vi "Zombie.vi"(8 "Error In":errorcluster, 11 "VI In":refnum<vi>) -> (0 "Error Out":errorcluster, 3 "VI Out":refnum<vi>)   [LabVIEW 2017, in "Eulogy.lvlib"]
uses:
  Eulogy.lvlib
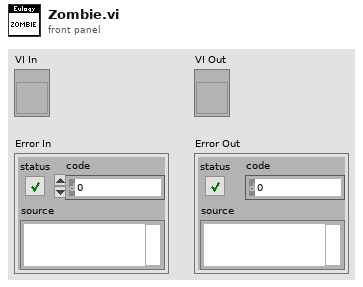
[diagram p1: front panel]
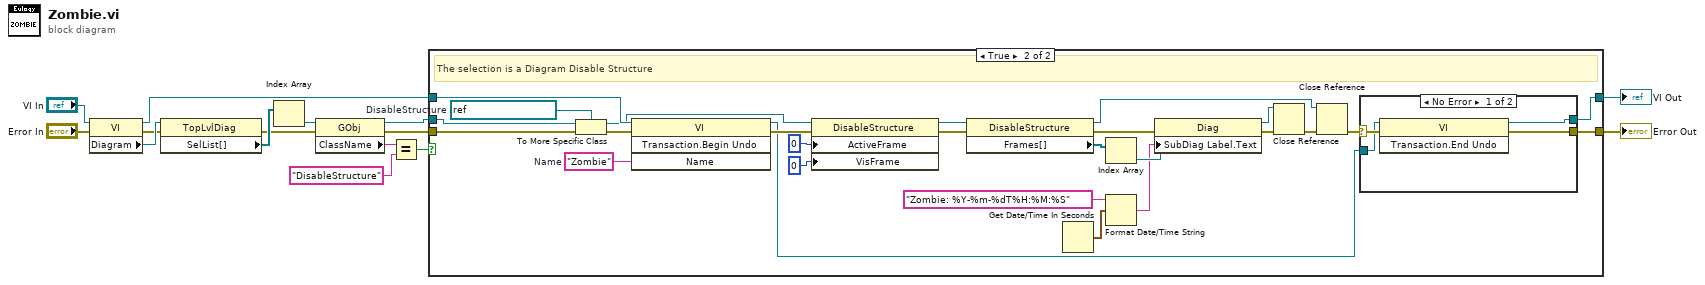
[diagram p0: block diagram]
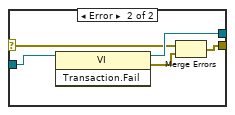
[diagram p3: hidden frame]
diagram:
  n1 = property class="VI"(reference="VI In", error in="Error In") -> (reference out=w7:refnum<vi>, error out=w12:errorcluster, "Diagram"=w13:refnum<vi>)
  n2 = property class="TopLvlDiag"(reference=w13, error in=w12) -> (error out=w9:errorcluster, "SelList[]"=w11:refnum<vi>[])  [unwired: 1 out]
  n3 = Index Array(array=w11) -> (element=w10:refnum<vi>)  [unwired: 1 in]
  n4 = property class="GObj"(reference=w10, error in=w9) -> (reference out=w2:refnum<vi>, error out=w1:errorcluster, "ClassName"=w5:string)
  n5 = Equal?(x=w5, y="DisableStructure") -> (x = y?=w3:bool)
  n6 = case shown="True" w3 {
    tunnel: [w16 w42] -> w15
    tunnel: [w17 w41] -> w14
    tunnel: w7 -> [w17 w40]
    tunnel: w2 -> [_ w38]
    tunnel: w1 -> [w16 w37]
    frame False {
      # "Selection is NOT a grave site, do nothing"
    }
    frame True {
      w39 = refnum<vi> refnum  # DisableStructure
      w43 = "Zombie"  # Name
      # "The selection is a Diagram Disable Structure"
      n7 = To More Specific Class(target class=w39, reference=w38, error in=w37) -> (specific class reference=w34:refnum<vi>, error out=w36:errorcluster)
      n8 = invoke class="VI" method="Transaction.Begin Undo"(reference=w40, error in=w36, "Name"=w43) -> (reference out=w31:refnum<vi>, error out=w35:errorcluster)  [unwired: 1 in, 2 out]
      n9 = property class="DisableStructure"(reference=w34, error in=w35, "ActiveFrame"=i16 0 ("Active Frame"), "VisFrame"=u32 0 ("Visible Frame")) -> (reference out=w29:refnum<vi>, error out=w28:errorcluster)
      n10 = property class="DisableStructure"(reference=w29, error in=w28) -> (reference out=w18:refnum<vi>, error out=w25:errorcluster, "Frames[]"=w27:refnum<vi>[])
      n11 = Get Date/Time In Seconds() -> (seconds since 1Jan1904=w24:timestamp)
      n12 = Index Array(array=w27) -> (element=w26:refnum<vi>)  [unwired: 1 in]
      n13 = Format Date/Time String(time format string (%c)="Zombie: %Y-%m-%dT%H:%M:%S", seconds (now)=w24) -> (date/time string=w22:string)  [unwired: 1 in]
      n14 = property class="Diag"(reference=w26, error in=w25, "SubDiag Label.Text"=w22) -> (reference out=w20:refnum<vi>, error out=w21:errorcluster)
      n15 = Close Reference(reference=w20, error in (no error)=w21) -> (error out=w19:errorcluster)
      n16 = Close Reference(reference=w18, error in (no error)=w19) -> (error out=w30:errorcluster)
      n17 = case shown="No Error" w30 {
        selector: w30 -> [w46 w49]
        tunnel: [w45 w50] -> w42
        tunnel: [w47 w52] -> w41
        tunnel: w31 -> [w44 w48]
        frame No Error {
          n18 = invoke class="VI" method="Transaction.End Undo"(reference=w44, error in=w46) -> (reference out=w47:refnum<vi>, error out=w45:errorcluster)  [unwired: 1 in, 1 out]
        }
        frame Error {
          n19 = invoke class="VI" method="Transaction.Fail"(reference=w48) -> (reference out=w52:refnum<vi>, error out=w51:errorcluster)  [unwired: 2 in, 1 out]
          n20 = Merge Errors(w49, w51) -> (w50:errorcluster)
        }
      }
    }
  }
  "Error Out" <- w15
  "VI Out" <- w14
